vi "Files to Post Process.vi"   [LabVIEW 2018]
uses:
  Controls/PP Raw data file cluster.ctl
  Globals/Meas_global.vi
  Globals/Trav_pos_global.vi
types:
  T1 = typedef "PP Raw data file cluster.ctl" = cluster{"Raw Data File":path, "Results File":path}
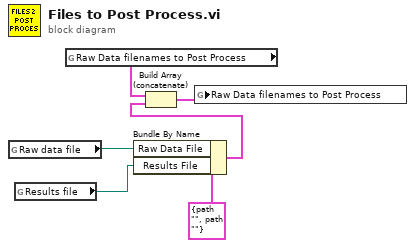
[diagram p0: block diagram]
diagram:
  n1 = global read "Meas_global.vi" "Raw data file"() -> (w3:path)
  n2 = global read "Meas_global.vi" "Results file"() -> (w4:path)
  n3 = global read "Trav_pos_global.vi" "Raw Data filenames to Post Process"() -> (w2:T1[])
  n4 = Bundle By Name(cluster=T1 {"Raw Data File"=path "", "Results File"=path ""} ("Cluster"), "Raw Data File"=w3, "Results File"=w4) -> (w6:T1)
  n5 = Build Array (concatenate)(w2, w6) -> (w1:T1[])
  n6 = global write "Trav_pos_global.vi" "Raw Data filenames to Post Process"(w1) -> ()
